vi "Start PJVS.vi"(8 "error in (pass through)":errorcluster, 10 "Measurement properties":T1={"Measurement ID"=enum."1", "Description"="3 phase, 3 ADC, 1 PJVS", "Switching matrix M"=[], "Signal frequency  (Hz)"=50.0, "Signal amplitudes (V)"=[], "PRs"=1, "PRe"=50, "MRs"=0, "MRe"=0, "Set PJVS frequency (Hz)"=50.0, "PJVS reference voltages (1 period, V)"=[], "Requiested PJVS steps"=10, "Sampling f (Hz)"=7000.0} {"PJVS reference voltages (1 period, V)" format="%.9g"}, 11 "PJVS setup":T3={"PJVS type"=enum."AC-supraVOLTcontrol", "Status Refnum"=refnum, "Abort Refnum"=refnum, "AC-supraVOLTcontrol"={"IP address:port (0.0.0.0:0000)"="0.0.0.0:0000", "Timeouts"={"TCP Read & Write (ms)"=7000, "Sensors readout"=5000, "PJVS setup"=10000, "Nullmeter readout"=5000, "Multiplexer setup"=3000, "57XX setup"=15000, "Generator setup"=5000, "Synthesizer setup"=3000, "Sampler readout"=10000}, "Simulation mode"=FALSE, "Debug mode"=FALSE}, "NPL bias source"={"DataSocketCluster"={"Server Machine"="CZC", "Client Machine"="localhost", "Data"="P2", "TimeStamp"=0.0, "Count"=1, "Target Process"="General Server"}}} {"NPL bias source"."DataSocketCluster"."TimeStamp" format="%.2f"}) -> (0 "error out":errorcluster, 2 "Measurement properties out":T1={"Measurement ID"=enum."1", "Description"="3 phase, 3 ADC, 1 PJVS", "Switching matrix M"=[], "Signal frequency  (Hz)"=50.0, "Signal amplitudes (V)"=[], "PRs"=1, "PRe"=10, "MRs"=0, "MRe"=0, "Set PJVS frequency (Hz)"=50.0, "PJVS reference voltages (1 period, V)"=[], "Requiested PJVS steps"=10, "Sampling f (Hz)"=7000.0} {"PJVS reference voltages (1 period, V)" format="%.9g"}, 3 "PJVS setup out":T3={"PJVS type"=enum."AC-supraVOLTcontrol", "Status Refnum"=refnum, "Abort Refnum"=refnum, "AC-supraVOLTcontrol"={"IP address:port (0.0.0.0:0000)"="0.0.0.0:0000", "Timeouts"={"TCP Read & Write (ms)"=7000, "Sensors readout"=5000, "PJVS setup"=10000, "Nullmeter readout"=5000, "Multiplexer setup"=3000, "57XX setup"=15000, "Generator setup"=5000, "Synthesizer setup"=3000, "Sampler readout"=10000}, "Simulation mode"=FALSE, "Debug mode"=FALSE}, "NPL bias source"={"DataSocketCluster"={"Server Machine"="CZC", "Client Machine"="localhost", "Data"="P2", "TimeStamp"=0.0, "Count"=1, "Target Process"="General Server"}}} {"NPL bias source"."DataSocketCluster"."TimeStamp" format="%.2f"})   [LabVIEW 2020]
doc: "Initialize the PJVS. Calls the initialization routine of the actual driver."
uses:
  Type definitions/PJVS Setup.ctl
  Type definitions/PJVS Type.ctl
  PJVS drivers/acsvcontrol-driver/build/ACSVcontrol-driver_0.2.0.0.llb/Timeouts.ctl
  PJVS drivers/JV modified NPL Bias source/DataSocketCluster external.ctl
  Measurement/Type definitions/Measuement properties.ctl
  Measurement/Type definitions/Measurement ID.ctl
  PJVS drivers/acsvcontrol-driver/build/ACSVcontrol-driver_0.2.0.0.llb/Waveform.ctl
  PJVS drivers/acsvcontrol-driver/build/ACSVcontrol-driver_0.2.0.0.llb/Multiplexer.ctl
  PJVS drivers/acsvcontrol-driver/build/ACSVcontrol-driver_0.2.0.0.llb/ACSVcontrol-driver.lvlib
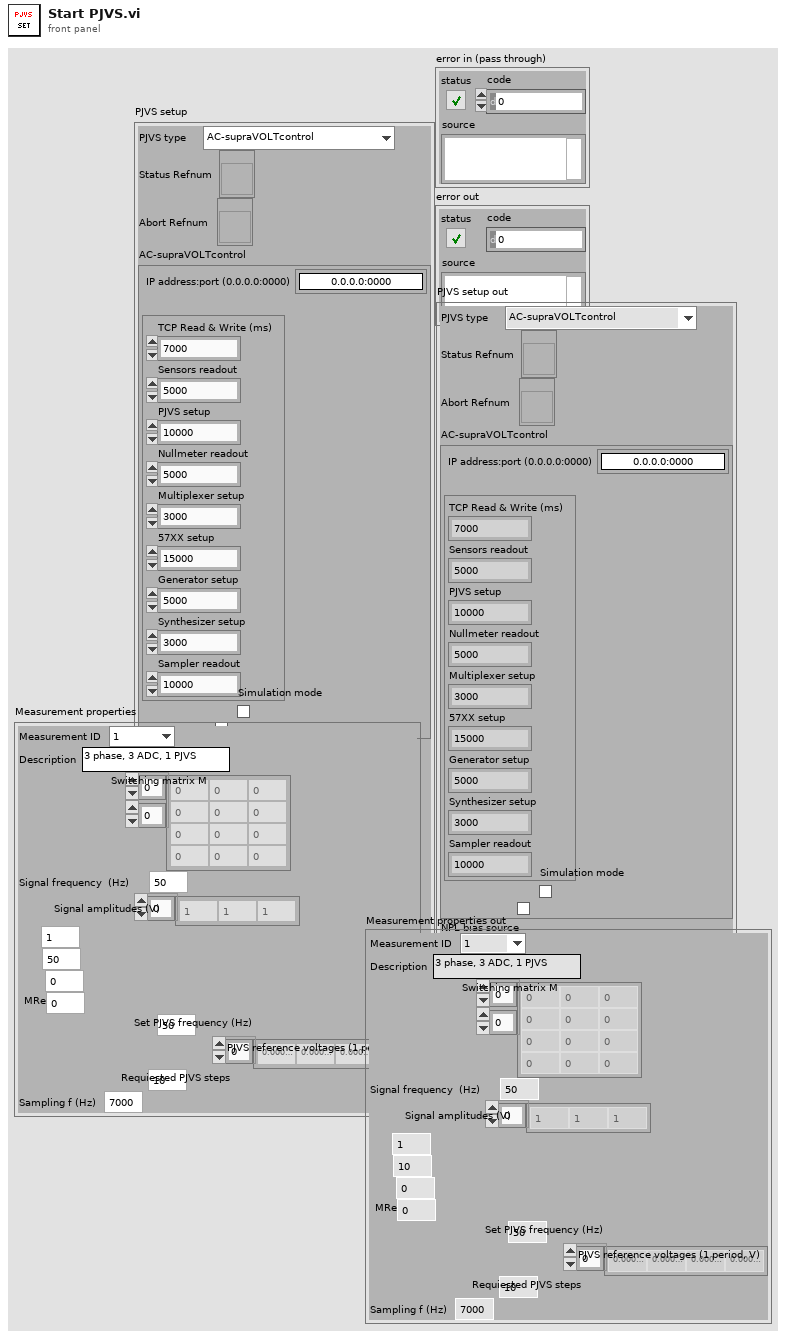
[diagram p1: front panel]
types:
  T1 = typedef "Measuement properties.ctl" = cluster{"Measurement ID":T2, "Description":string, "Switching matrix M":i32[][], "Signal frequency  (Hz)":dbl, "Signal amplitudes (V)":dbl[], "PRs":i32, "PRe":i32, "MRs":i32, "MRe":i32, "Set PJVS frequency (Hz)":dbl, "PJVS reference voltages (1 period, V)":dbl[], "Requiested PJVS steps":i32, "Sampling f (Hz)":dbl}
  T2 = typedef "Measurement ID.ctl" = enum16{"M", "1", "2", "3"}
  T3 = typedef "PJVS Setup.ctl" = cluster{"PJVS type":T4, "Status Refnum":refnum<vi>, "Abort Refnum":refnum<vi>, "AC-supraVOLTcontrol":cluster{"IP address:port (0.0.0.0:0000)":string, "Timeouts":T5, "Simulation mode":bool, "Debug mode":bool}, "NPL bias source":cluster{"DataSocketCluster":T6}}
  T4 = typedef "PJVS Type.ctl" = enum16{"AC-supraVOLTcontrol", "JV modified NPL bias control"}
  T5 = typedef "ACSVcontrol-driver.lvlib/Timeouts.ctl" = cluster{"TCP Read & Write (ms)":i32, "Sensors readout":i32, "PJVS setup":i32, "Nullmeter readout":i32, "Multiplexer setup":i32, "57XX setup":i32, "Generator setup":i32, "Synthesizer setup":i32, "Sampler readout":i32}
  T6 = typedef "DataSocketCluster external.ctl" = cluster{"Server Machine":string, "Client Machine":string, "Data":string, "TimeStamp":dbl, "Count":i32, "Target Process":string}
  T7 = typedef "ACSVcontrol-driver.lvlib/Multiplexer.ctl" = enum16{"Short DC Nano / Voltmeter", "Short AC Sampler", "Short Switch DC (JVS->Nano)", "Short Switch AC (JVS->Digit)", "JVS-Voltmeter", "Channel A positive", "Channel A negative", "Channel B positive", "Channel B negative", "Channel C positive", "Channel C negative", "Nulldetector-Channel A+", "Nulldetector-Channel A-", "Nulldetector-Channel B+", "Nulldetector-Channel B-", "Nulldetector-Channel C+", "Nulldetector-Channel C-", "ext.Voltmeter-Channel A+", "ext.Voltmeter-Channel A-", "ext.Voltmeter-Channel B+", "ext.Voltmeter-Channel B-", "ext.Voltmeter-Channel C+", "ext.Voltmeter-Channel C-"}
  T8 = typedef "ACSVcontrol-driver.lvlib/Waveform.ctl" = enum16{"Sinewave", "Triangle", "Sawtooth", "Rectangle", "Arbitrary"}
  T9 = typedef "ACSVcontrol-driver.lvlib/PJVS Voltages.ctl" = cluster{"DC Voltage (S)":dbl, "AC Josephson Voltage RMS (V)":dbl, "Number of steps":i32, "AC Voltages (V)":dbl[]}
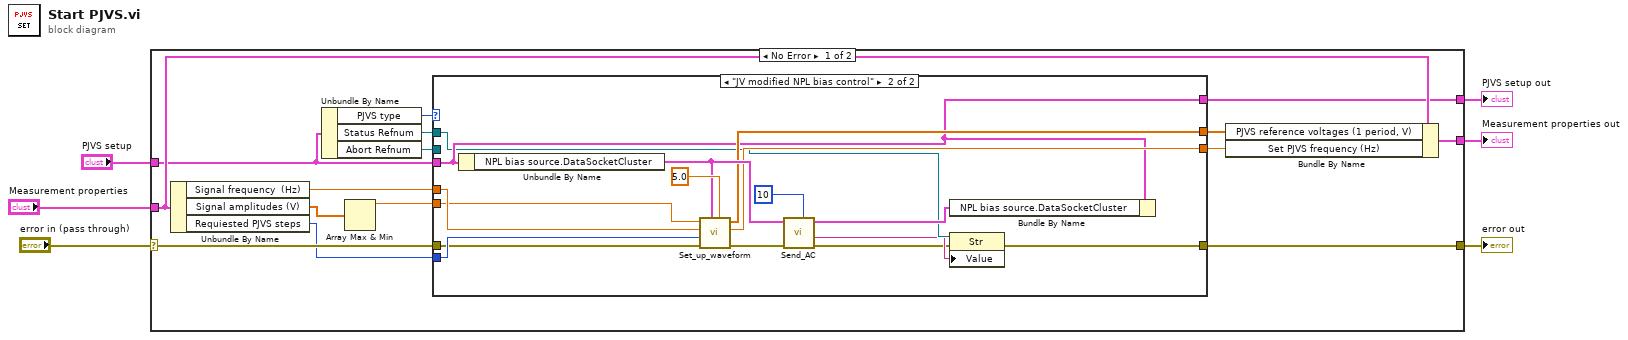
[diagram p0: block diagram]
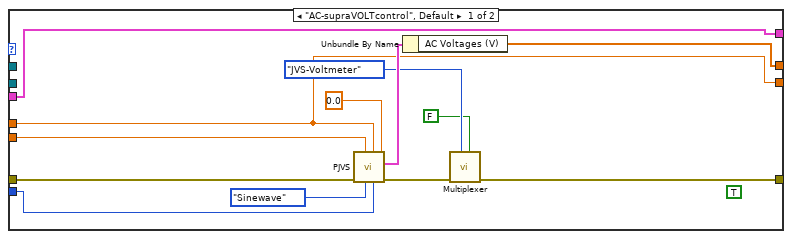
[diagram p2: hidden frame]
diagram:
  n1 = case shown="No Error" "error in (pass through)" {
    selector: "error in (pass through)" -> [w17 w53]
    tunnel: "PJVS setup" -> [w8 w52]
    tunnel: [w18 w53] -> w5
    tunnel: [w7 w52] -> w3
    tunnel: "Measurement properties" -> [w10 w51]
    tunnel: [w13 w51] -> w1
    frame No Error {
      n2 = Unbundle By Name(w10) -> ("Signal frequency  (Hz)"=w16:dbl, "Signal amplitudes (V)"=w12:dbl[], "Requiested PJVS steps"=w15:i32)
      n3 = Unbundle By Name(w8) -> ("PJVS type"=w21:T4, "Status Refnum"=w20:refnum<vi>, "Abort Refnum"=w19:refnum<vi>)
      n4 = Array Max & Min(array=w12) -> (max value=w11:dbl)  [unwired: 3 out]
      n5 = case shown="\"JV modified NPL bias control\"" w21 {
        tunnel: w20 -> [_ w40]
        tunnel: w19 -> [_ _]
        tunnel: w17 -> [w34 w38]
        tunnel: [w24 w35] -> w18
        tunnel: w16 -> [w23 w48]
        tunnel: w11 -> [w31 w46]
        tunnel: w15 -> [w30 w47]
        tunnel: [w28 w45] -> w14
        tunnel: w8 -> [w22 w42]
        tunnel: [w23 w44] -> w9
        tunnel: [w22 w42] -> w7
        frame "AC-supraVOLTcontrol", Default {
          (unwired) TRUE ("Waveform (F) (F:Sine, T:Square)")
          n6 = call "PJVS.vi"("Trim current (A) (+- 0.002)"=0.0, "Samples (2) (2 - 256)"=w30, "Frequency  (0 Hz) (0, 0.5 - 10e3)"=w23, "Waveform (Sinewave)"=Waveform."Sinewave", "Voltage (0 V DC/RMS) (DC: +- 10.1, AC: 0 - 7.2)"=w31, "error in (no error)"=w34) -> ("error out"=w27:errorcluster, "PJVS Voltages"=w29:T9)  [unwired: 4 in]
          n7 = Unbundle By Name(w29) -> ("AC Voltages (V)"=w28:dbl[])
          n8 = call "Multiplexer.vi"("AC (F) (F:Nano, T:Digitizer)"=FALSE, "Multiplexer (Short DC Nano / Voltmeter)"=Multiplexer."JVS-Voltmeter", "error in (no error)"=w27) -> ("error out"=w24:errorcluster)  [unwired: 8 in]
        }
        frame "JV modified NPL bias control" {
          n9 = Unbundle By Name(w42) -> ("NPL bias source.DataSocketCluster"=w49:T6)
          n10 = call "Set_up_waveform.vi"("TimeOut Time (s)"=5.0, "DataSocketCluster In"=w49, "error in (no error)"=w38, "Steps on PJVS curve"=w47, "Frequency (Hz)"=w48, "Amplitude (V)"=w46) -> ("error IO"=w37:errorcluster, "Set frequency (Hz)"=w44:dbl, "Voltage at each step on PJVS curve"=w45:dbl[])  [unwired: 3 out]
          n11 = call "Send_AC.vi"("milliseconds to wait"=u32 10, "error in (no error)"=w37, "DataSocketCluster In"=w49) -> ("error out"=w36:errorcluster, "Response to SEND AC"=w39:string, "DataSocketCluster out"=w41:T6)  [unwired: 6 in]
          n12 = Bundle By Name(cluster=w42, "NPL bias source.DataSocketCluster"=w41) -> ()  [unwired: 1 out]
          n13 = property class="Str"(reference=w40, error in=w36, "Value"=w39) -> (error out=w35:errorcluster)  [unwired: 1 out]
        }
      }
      n14 = Bundle By Name(cluster=w10, "PJVS reference voltages (1 period, V)"=w14, "Set PJVS frequency (Hz)"=w9) -> (w13:T1)
    }
    frame Error {
    }
  }
  "error out" <- w5
  "PJVS setup out" <- w3
  "Measurement properties out" <- w1
